vi "ma_design Kaiser windowed FIR filter.vi"(7 "error in":errorcluster, 10 "FIR filter specifications":T1={"alias rejection (dB)"=125.0, "normalized bandwidth"=0.4536} {"normalized bandwidth" format="%.4f"; "alias rejection (dB)" format="%.2f"}) -> (0 "error out":errorcluster, 3 "filter data":cluster{"h":dbl[], "Max Decimation":dbl}={"h"=[], "Max Decimation"=1024.0} {"Max Decimation" format="%.2f"; "h" format="%.2p"})   [LabVIEW 2020, in "NI_MAPro.lvlib"]
uses:
  NI_MAPro.lvlib
  NI_AALBase.lvlib
  NI_AALPro.lvlib
  NI_MABase.lvlib
panel:
  out "Waveform Graph":dbl[](graph)
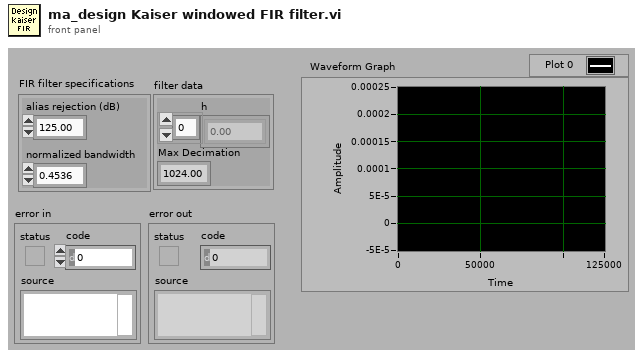
[diagram p1: front panel]
types:
  T1 = cluster{"alias rejection (dB)":dbl, "normalized bandwidth":dbl}
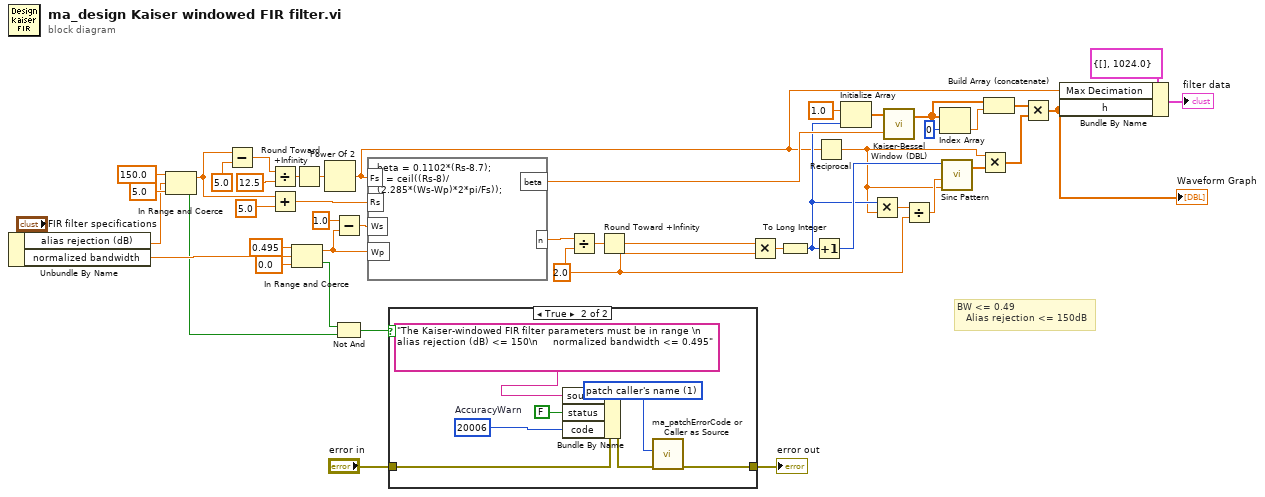
[diagram p0: block diagram]
diagram:
  w28 = 2.0 ("y")
  # "BW <= 0.49\n   Alias rejection <= 150dB"
  n1 = Unbundle By Name("FIR filter specifications") -> ("alias rejection (dB)"=w7:dbl, "normalized bandwidth"=w13:dbl)
  n2 = In Range and Coerce(upper limit=150.0, x=w7, lower limit=5.0) -> (coerced(x)=w8:dbl, In Range?=w5:bool)
  n3 = Subtract(x=w8, y=5.0) -> (x-y=w19:dbl)
  n4 = Divide(x=w19, y=12.5) -> (x/y=w18:dbl)
  n5 = Add(x=w8, y=5.0) -> (x+y=w17:dbl)
  n6 = In Range and Coerce(upper limit=0.495, x=w13, lower limit=0.0) -> (coerced(x)=w14:dbl, In Range?=w6:bool)
  n7 = Round Toward +Infinity(x=w18) -> (ceil(x): smallest int >= x=w25:dbl)
  n8 = Power Of 2(x=w25) -> (2^x=w22:dbl)
  n9 = Subtract(x=1.0, y=w14) -> (x-y=w26:dbl)
  n10 = Not And(1:w5, 2:w6) -> (0:w4:bool)
  n11 = formula code="beta = 0.1102*(Rs-8.7);\nn = ceil((Rs-8)/(2.285*(Ws-Wp)*2*pi/Fs));"("Rs"=w17, "Ws"=w26, "Wp"=w14, "Fs"=w22) -> ("beta"=w46:dbl, "n"=w40:dbl)
  n12 = case shown="True" w4 {
    tunnel: "error in" -> [w47 w49]
    tunnel: [w47 w48] -> w2
    frame False {
    }
    frame True {
      w51 = u16 1 items=["patch error code", "patch caller's name"] ("operation")
      w52 = 20006  # AccuracyWarn
      n13 = Bundle By Name(cluster=w49, "source"="The Kaiser-windowed FIR filter parameters must be in range \n     alias rejection (dB) <= 150\n     normalized bandwidth <= 0.495" ("initial string"), "status"=FALSE, "code"=w52) -> (w50:errorcluster)
      n14 = call "ma_patchErrorCode or Caller as Source.vi"("error in (no error)"=w50, "operation"=w51) -> ("error out"=w48:errorcluster)  [unwired: 9 in]
    }
  }
  "error out" <- w2
  n15 = Divide(x=w40, y=w28) -> (x/y=w38:dbl)
  n16 = Round Toward +Infinity(x=w38) -> (ceil(x): smallest int >= x=w37:dbl)
  n17 = Multiply(x=w37, y=w28) -> (x*y=w39:dbl)
  n18 = To Long Integer(number=w39) -> (32bit integer=w31:i32)
  n19 = Increment(x=w31) -> (x+1=w36:i32)
  n20 = Reciprocal(x=w22) -> (1/x=w30:dbl)
  n21 = Initialize Array(1.0 ("Element Data"), w31) -> (w45:dbl[])
  n22 = Multiply(x=w31, y=w30) -> (x*y=w35:dbl)
  n23 = call "Kaiser-Bessel Window (DBL).vi"("beta"=w46, "X"=w45) -> ("Windowed X"=w43:dbl[])  [unwired: 1 out]
  n24 = Divide(x=w35, y=w28) -> (x/y=w34:dbl)
  n25 = Index Array(array=w43, index=0 ("Index")) -> (element=w42:dbl)
  n26 = call "Sinc Pattern.vi"("delta t"=w30, "delay"=w34, "samples"=w36) -> ("Sinc Pattern"=w29:dbl[])  [unwired: 1 in, 1 out]
  n27 = Multiply(x=w30, y=w29) -> (x*y=w33:dbl[])
  n28 = Build Array (concatenate)(w43, w42) -> (w32:dbl[])
  n29 = Multiply(x=w32, y=w33) -> (x*y=w1:dbl[])
  "Waveform Graph" <- w1
  n30 = Bundle By Name(cluster=cluster{"h":dbl[], "Max Decimation":dbl} {"h"=[], "Max Decimation"=1024.0} ("filter old"), "Max Decimation"=w22, "h"=w1) -> (→"filter data":cluster{"h":dbl[], "Max Decimation":dbl})
